vi "Teleop.vi"(10 "Match Info":T1={"Autonomous Elapsed Seconds"=0.0, "TeleOp Elapsed Seconds"=0.0, "Disabled Elapsed Seconds"=0.0, "Visited Autonomous"=FALSE, "Visited TeleOp"=FALSE, "Visited Disabled"=FALSE, "Autonomous Settings"={"Autonomous Style"=enum."Independent", "VI Refnum"=refnum}}, 11 "Call Context":T2) -> ()   [LabVIEW 2015]
doc: "This VI is called for each TeleOp packet received from the DS where the robot is not disabled. It is often used to read from the joysticks and update I/O or to update setpoints for timed control loops. It should complete and return within 20 milliseconds or it may miss DS packets."
uses:
  <vilib>/Rock Robotics/WPI/DriverStation/WPI_DriverStationDerivedRobotMode.ctl
  <vilib>/Rock Robotics/WPI/DriverStation/WPI_DriverStationMatch Info.ctl
  <vilib>/Rock Robotics/Network Tables/NT Read Boolean.vi
  <vilib>/Rock Robotics/Network Tables/NT Read Number.vi
  <vilib>/Rock Robotics/WPI/Utilities/WPI_GetSetVariantRefNum.vi
  <vilib>/Rock Robotics/Network Tables/SD Write Number.vi
  <vilib>/Rock Robotics/Network Tables/NT Write Number.vi
  navX Library v2/navX Library v2.lvlib
  <vilib>/Rock Robotics/Network Tables/NT Write Boolean.vi
panel:
  out "Displacement X":dbl
  out "Velocity X":dbl
  out "Sample Slider 0":dbl(slide) scale=0.0..5.0
  out "Sample Boolean 1":bool
  out "Sample Boolean 0":bool
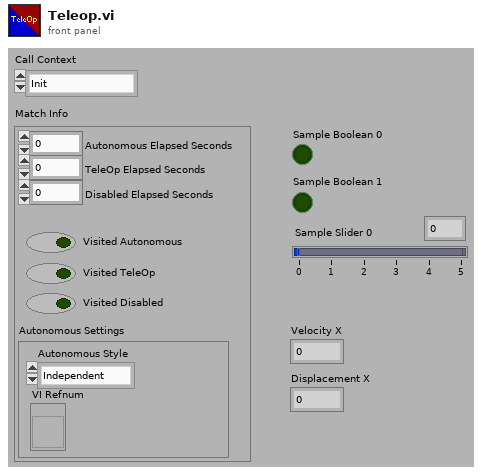
[diagram p1: front panel]
types:
  T1 = typedef "WPI_DriverStationMatch Info.ctl" = cluster{"Autonomous Elapsed Seconds":dbl, "TeleOp Elapsed Seconds":dbl, "Disabled Elapsed Seconds":dbl, "Visited Autonomous":bool, "Visited TeleOp":bool, "Visited Disabled":bool, "Autonomous Settings":cluster{"Autonomous Style":enum16{"Iterative", "Independent"}, "VI Refnum":refnum<vi>}}
  T2 = typedef "WPI_DriverStationDerivedRobotMode.ctl" = enum16{"Init", "Execute", "Stop"}
  T3 = typedef "navX Library v2.lvlib/Z900_navX_DeviceTypeDef.ctl" = cluster{"Interface":cluster{"Protocol":T4, "Update Rate (4Hz-60Hz)":u8, "navX Open TypeDef":variant}, "Notify Packet":refnum<notifier>, "Loop VI Refnum":refnum<vi>, "Ready to Close Occurrence Refnum":refnum<k4>}
  T4 = typedef "navX Library v2.lvlib/Z900_navX_ProtocolTypeDef.ctl" = enum16{"SERIAL", "I2C", "SPI"}
  T5 = typedef "WPI_EncoderDevRef.ctl" = cluster{"DevStatus":errorcluster, "EncoderIndex":T6, "CounterIndex":T7, "DistancePerCount":dbl, "Decoding Type":T8}
  T6 = typedef "FPGA_EncoderIdx.ctl" = enum8{"Enc 0", "Enc 1", "Enc 2", "Enc 3", "Enc 4", "Enc 5", "Enc 6", "Enc 7", "Invalid"}
  T7 = typedef "FPGA_CounterCtrSystemIndex.ctl" = enum8{"Ctr 0", "Ctr 1", "Ctr 2", "Ctr 3", "Ctr 4", "Ctr 5", "Ctr 6", "Ctr 7", "Invalid"}
  T8 = typedef "WPI_EncoderType.ctl" = enum16{"1x", "2x", "4x"}
  T9 = typedef "WPI_JoystickDevRef.ctl" = cluster{"Device":T10}
  T10 = typedef "WPI_JoystickDeviceEnum.ctl" = enum16{"USB 0", "USB 1", "USB 2", "USB 3", "USB 4", "USB 5"}
  T11 = cluster{"Velocity X":dbl, "Velocity Y":dbl, "Velocity Z":dbl, "Displacement X":dbl, "Displacement Y":dbl, "Displacement Z":dbl}
  T12 = cluster{"LinearAcceleration X":dbl, "LinearAcceleration Y":dbl, "LinearAcceleration Z":dbl}
  T13 = cluster{"Yaw":dbl, "Roll":dbl, "Pitch":dbl, "Heading":dbl, "Fused Heading":dbl}
  T14 = cluster{"Axes[0]":dbl, "Axes[1]":dbl, "Axes[2]":dbl, "Axes[3]":dbl, "Axes[4]":dbl, "Axes[5]":dbl, "Axes[6]":dbl, "Axes[7]":dbl, "Axes[8]":dbl}
  T15 = cluster{"Buttons[0]":bool, "Buttons[1]":bool, "Buttons[2]":bool, "Buttons[3]":bool, "Buttons[4]":bool, "Buttons[5]":bool, "Buttons[6]":bool, "Buttons[7]":bool, "Buttons[8]":bool}
  T16 = typedef "WPI_RobotDriveDevRef.ctl" = cluster{"DevStatus":errorcluster, "Motors[]":T17[], "Square Inputs":bool, "Max Output":dbl}
  T17 = typedef "WPI_MotorControlDeviceRef.ctl" = cluster{"DeviceStatus":errorcluster, "Type":T18, "PWM":cluster{"PWM Channel":T19, "DeadBand":T20}, "CAN":cluster{"Device Number":u8, "Control Mode":T21, "Semaphore":T22, "Max Vout":dbl, "TalonSRX Control Mode":T23}, "Invert":bool}
  T18 = typedef "WPI_MotorControlType.ctl" = enum16{"PWM", "CAN", "CANTalonSRX"}
  T19 = typedef "FPGA_DIOPWMChannel.ctl" = enum8{"PWM 0", "PWM 1", "PWM 2", "PWM 3", "PWM 4", "PWM 5", "PWM 6", "PWM 7", "PWM 8", "PWM 9", "PWM MXP 0", "PWM MXP 1", "PWM MXP 2", "PWM MXP 3", "PWM MXP 4", "PWM MXP 5", "PWM MXP 6", "PWM MXP 7", "PWM MXP 8", "PWM MXP 9", "Invalid"}
  T20 = typedef "WPI_PWMDeadband.ctl" = cluster{"Name":string, "maxPositivePwm":i32, "minPositivePwm":i32, "centerPwm":i32, "maxNegativePwm":i32, "minNegativePwm":i32, "angularRange":u16}
  T21 = typedef "WPI_CANJaguar_ControlMode.ctl" = enum8{"Percent VBus", "Current", "Speed", "Position", "Voltage"}
  T22 = typedef "Semaphore RefNum" = refnum<k1>
  T23 = typedef "WPI_CANTalonSRX_APIControlMode.ctl" = enum8{"Percent VBus", "Speed", "Position", "Slave", "Unchanged / Invalid", "Voltage Compensation", "Current", "Motion Profile"}
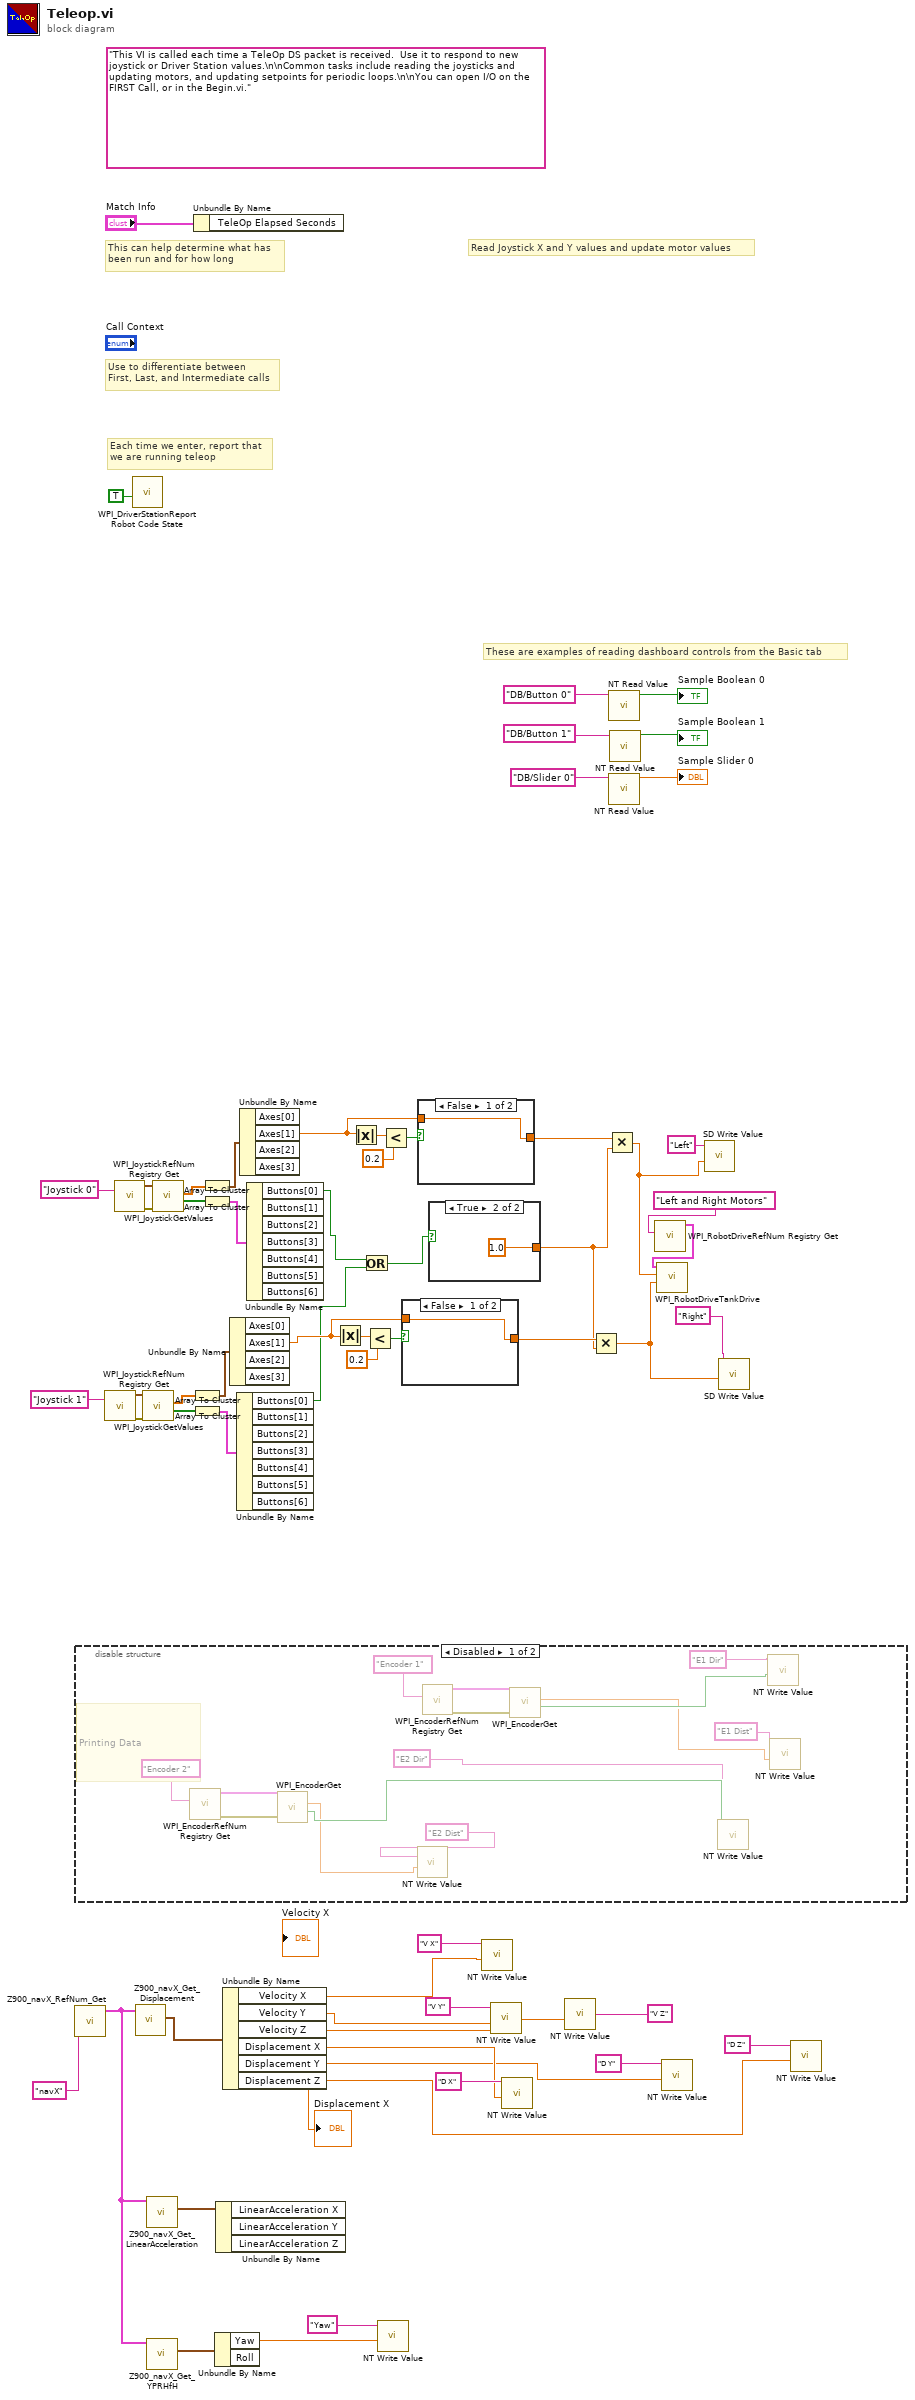
[diagram p0: block diagram]
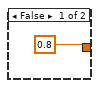
[diagram p3: hidden frame]
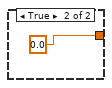
[diagram p4: hidden frame]
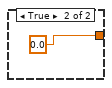
[diagram p5: hidden frame]
diagram:
  (unwired) "This VI is called each time a TeleOp DS packet is received.  Use it to respond to new joystick or Driver Station values.\n\nCommon tasks include reading the joysticks and updating motors, and updating setpoints for periodic loops.\n\nYou can open I/O on the FIRST Call, or in the Begin.vi."
  # "These are examples of reading dashboard controls from the Basic tab"
  # "Each time we enter, report that\nwe are running teleop"
  # "Use to differentiate between\nFirst, Last, and Intermediate calls"
  # "This can help determine what has\nbeen run and for how long"
  # "Read Joystick X and Y values and update motor values"
  n1 = call "Z900_navX_RefNum_Get.vi"("refnum name"="navX") -> ("navX Device"=w4:T3)  [unwired: 9 in, 1 out]
  n2 = disable-structure shown="Disabled" {
    frame Disabled {
      # "Printing Data"
      n3 = call <vilib>:"WPI_EncoderRefNum Registry Get.vi"("refnum name"="Encoder 2") -> ("error out"=w71:errorcluster, "EncoderDevRef"=w70:T5)  [unwired: 9 in]
      n4 = call <vilib>:"WPI_EncoderGet.vi"("error in (no error)"=w71, "EncoderDevRef"=w70) -> ("Direction"=w65:bool, "Distance"=w62:dbl)  [unwired: 4 in, 4 out]
      n5 = call-poly <vilib>:"NT Write Value.vi"("Numeric"=w62, "Name"="E2 Dist") -> ()  [unwired: 9 in, 1 out]
      n6 = call <vilib>:"WPI_EncoderRefNum Registry Get.vi"("refnum name"="Encoder 1") -> ("error out"=w74:errorcluster, "EncoderDevRef"=w73:T5)  [unwired: 9 in]
      n7 = call <vilib>:"WPI_EncoderGet.vi"("error in (no error)"=w74, "EncoderDevRef"=w73) -> ("Direction"=w68:bool, "Distance"=w66:dbl)  [unwired: 4 in, 4 out]
      n8 = call-poly <vilib>:"NT Write Value.vi"("Boolean"=w65, "Name"="E2 Dir") -> ()  [unwired: 9 in, 1 out]
      n9 = call-poly <vilib>:"NT Write Value.vi"("Boolean"=w68, "Name"="E1 Dir") -> ()  [unwired: 9 in, 1 out]
      n10 = call-poly <vilib>:"NT Write Value.vi"("Numeric"=w66, "Name"="E1 Dist") -> ()  [unwired: 9 in, 1 out]
    }
    frame Enabled {
    }
  }
  n11 = call <vilib>:"WPI_JoystickRefNum Registry Get.vi"("refnum name"="Joystick 1") -> ("error out"=w45:errorcluster, "JoystickDevRef"=w44:T9)  [unwired: 9 in]
  n12 = call <vilib>:"WPI_JoystickRefNum Registry Get.vi"("refnum name"="Joystick 0") -> ("error out"=w52:errorcluster, "JoystickDevRef"=w51:T9)  [unwired: 9 in]
  n13 = call <vilib>:"WPI_DriverStationReport Robot Code State.vi"("TeleOp"=TRUE ("Autonomous")) -> ()  [unwired: 10 in, 1 out]
  n14 = call "Z900_navX_Get_Displacement.vi"("navX Device"=w4) -> ("Displacement"=w19:T11)  [unwired: 7 in, 3 out]
  n15 = call <vilib>:"WPI_JoystickGetValues.vi"("error in (no error)"=w45, "JoystickDevRef"=w44) -> ("Buttons"=w42:bool[], "Axes"=w43:dbl[])  [unwired: 5 in, 3 out]
  n16 = call "Z900_navX_Get_LinearAcceleration.vi"("navX Device"=w4) -> ("Linear Acceleration"=w11:T12)  [unwired: 7 in, 3 out]
  n17 = call "Z900_navX_Get_YPRHfH.vi"("navX Device"=w4) -> ("YRPHfH"=w3:T13)  [unwired: 7 in, 3 out]
  n18 = call <vilib>:"WPI_JoystickGetValues.vi"("error in (no error)"=w52, "JoystickDevRef"=w51) -> ("Buttons"=w49:bool[], "Axes"=w50:dbl[])  [unwired: 5 in, 3 out]
  n19 = Array To Cluster(array=w43) -> (cluster=w41:T14)
  n20 = Array To Cluster(array=w42) -> (cluster=w40:T15)
  n21 = Unbundle By Name("Match Info") -> ()  [unwired: 1 out]
  n22 = Array To Cluster(array=w50) -> (cluster=w48:T14)
  n23 = Array To Cluster(array=w49) -> (cluster=w47:T15)
  n24 = Unbundle By Name(w3) -> ("Yaw"=w1:dbl)  [unwired: 1 out]
  n25 = Unbundle By Name(w11) -> ()  [unwired: 3 out]
  n26 = Unbundle By Name(w19) -> ("Velocity X"=w17:dbl, "Velocity Y"=w15:dbl, "Velocity Z"=w12:dbl, "Displacement X"=w7:dbl, "Displacement Y"=w6:dbl, "Displacement Z"=w5:dbl)
  "Displacement X" <- w7
  n27 = Unbundle By Name(w41) -> ("Axes[1]"=w30:dbl)  [unwired: 3 out]
  n28 = Unbundle By Name(w40) -> ("Buttons[0]"=w22:bool)  [unwired: 6 out]
  n29 = Unbundle By Name(w48) -> ("Axes[1]"=w35:dbl)  [unwired: 3 out]
  n30 = Unbundle By Name(w47) -> ("Buttons[0]"=w23:bool)  [unwired: 6 out]
  n31 = Absolute Value(x=w30) -> (abs(x)=w34:dbl)
  n32 = Absolute Value(x=w35) -> (abs(x)=w39:dbl)
  n33 = Or(x=w23, y=w22) -> (x .or. y?=w21:bool)
  n34 = Less?(x=w34, y=0.2) -> (x < y?=w32:bool)
  n35 = call-poly <vilib>:"NT Write Value.vi"("Numeric"=w1, "Name"="Yaw") -> ()  [unwired: 9 in, 1 out]
  n36 = Less?(x=w39, y=0.2) -> (x < y?=w37:bool)
  n37 = case shown="False" w32 {
    tunnel: [w76 0.0] -> w31
    tunnel: w30 -> [w76 _]
    frame False {
    }
    frame True {
    }
  }
  n38 = case shown="False" w37 {
    tunnel: [w78 0.0] -> w36
    tunnel: w35 -> [w78 _]
    frame False {
    }
    frame True {
    }
  }
  n39 = case shown="True" w21 {
    tunnel: [0.8 1.0] -> w29
    frame False {
    }
    frame True {
    }
  }
  n40 = call-poly <vilib>:"NT Write Value.vi"("Numeric"=w17, "Name"="V X") -> ()  [unwired: 9 in, 1 out]
  n41 = call-poly <vilib>:"NT Write Value.vi"("Numeric"=w15, "Name"="V Y") -> ()  [unwired: 9 in, 1 out]
  n42 = call-poly <vilib>:"NT Write Value.vi"("Numeric"=w7, "Name"="D X") -> ()  [unwired: 9 in, 1 out]
  n43 = call-poly <vilib>:"NT Write Value.vi"("Numeric"=w12, "Name"="V Z") -> ()  [unwired: 9 in, 1 out]
  n44 = Multiply(x=w31, y=w29) -> (x*y=w25:dbl)
  n45 = Multiply(x=w36, y=w29) -> (x*y=w24:dbl)
  n46 = call-poly <vilib>:"NT Read Value.vi"("Name"="DB/Button 0" ("refnum name")) -> ("Boolean"=→"Sample Boolean 0":bool)  [unwired: 9 in, 1 out]
  n47 = call-poly <vilib>:"NT Read Value.vi"("Name"="DB/Slider 0" ("refnum name")) -> ("Numeric"=→"Sample Slider 0":dbl)  [unwired: 9 in, 1 out]
  n48 = call-poly <vilib>:"NT Read Value.vi"("Name"="DB/Button 1" ("refnum name")) -> ("Boolean"=→"Sample Boolean 1":bool)  [unwired: 9 in, 1 out]
  n49 = call <vilib>:"WPI_RobotDriveRefNum Registry Get.vi"("refnum name"="Left and Right Motors") -> ("RobotDriveDevRef"=w28:T16)  [unwired: 9 in, 1 out]
  n50 = call <vilib>:"WPI_RobotDriveTankDrive.vi"("Right axis value"=w25, "Left axis value"=w24, "RobotDriveDevRef"=w28) -> ()  [unwired: 6 in, 3 out]
  n51 = call-poly <vilib>:"NT Write Value.vi"("Numeric"=w6, "Name"="D Y") -> ()  [unwired: 9 in, 1 out]
  n52 = call-poly <vilib>:"SD Write Value.vi"("Numeric"=w24, "Name"="Left") -> ()  [unwired: 8 in, 2 out]
  n53 = call-poly <vilib>:"SD Write Value.vi"("Numeric"=w25, "Name"="Right") -> ()  [unwired: 8 in, 2 out]
  n54 = call-poly <vilib>:"NT Write Value.vi"("Numeric"=w5, "Name"="D Z") -> ()  [unwired: 9 in, 1 out]
